vi "ExSubNframeColAdvDisp.vi"(0 "Handle Cluster":T1, 1 "SITKFULLDISPLAYLib.SITKFullDisplay":refnum<k7>, 2 "Number of Images":u32=1 min=1 step=1, 3 "error in (no error)":errorcluster) -> (4 "Handle Cluster":T1, 5 "error out":errorcluster)   [LabVIEW 2010]
panel:
  # "ExSubNframeColAdvDisp:\nThis is a sub VI that collects N frames from the camera\nsystem. This assumes camera has been setup and \ninitialized and that the start camera is done. It also \nassumes the camera has circular buffer capabillities.\nThis is not true for all cameras."
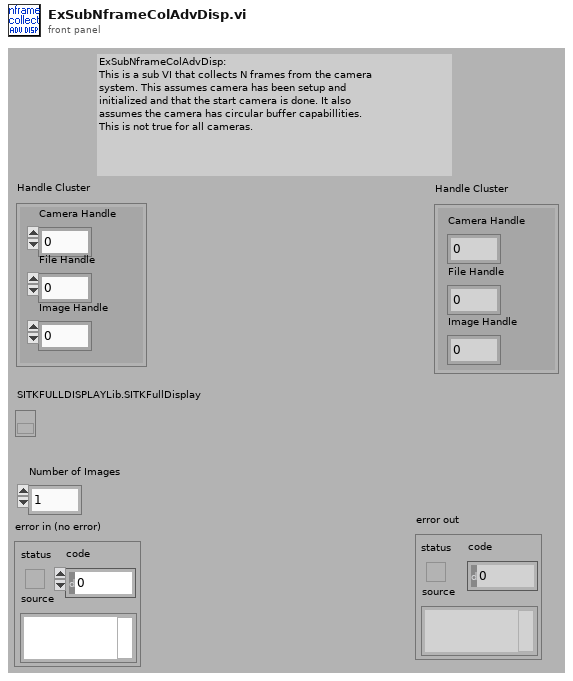
[diagram p1: front panel]
types:
  T1 = cluster{"Camera Handle":u32, "File Handle":u32, "Image Handle":u32}
  T2 = cluster{i32, "X dimension":u32, i32, "Y dimension":u32}
  T3 = cluster{"Min Value":dbl, "Min X Pos":u32, "Min Y Pos":u32, "Max Value":dbl, "Max X Pos":u32, "Max Y Pos":u32, "Reserved 1":dbl, "Reserved2":u32, "Reserved3":u32, "Mean Value":dbl, "StdDev":dbl, "Variance":dbl, "Centroid X":dbl, "Centroid Y":dbl, "Total Area":dbl}
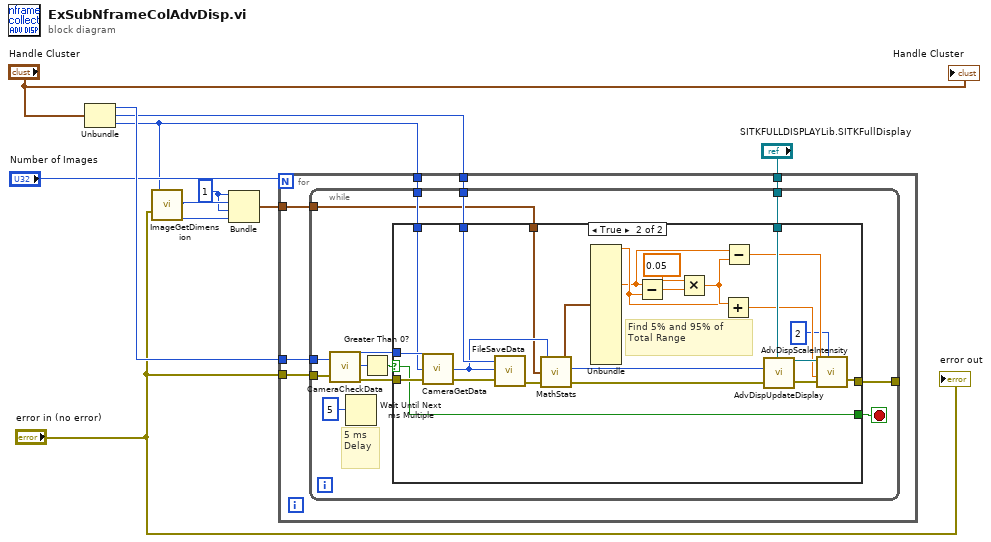
[diagram p0: block diagram]
diagram:
  w1 = 1
  n1 = Unbundle("Handle Cluster") -> ("Camera Handle"=w11:u32, "File Handle"=w6:u32, "Image Handle"=w5:u32)
  n2 = call <userlib>:"ImageGetDimension.vi"("Image Handle"=w5, "error in"="error in (no error)") -> ("X dimension"=w2:u32, "Y dimension"=w7:u32)  [unwired: 4 out]
  n3 = Bundle(w1, "X dimension"=w2, w1, "Y dimension"=w7) -> (w3:T2)  [unwired: 1 in]
  n4 = for {
    N: "Number of Images" -> [_]
    tunnel: w11 -> [w17]
    tunnel: "error in (no error)" -> [w16]
    tunnel: w5 -> [w15]
    tunnel: "SITKFULLDISPLAYLib.SITKFullDisplay" -> [w14]
    tunnel: w6 -> [w13]
    tunnel: w3 -> [w12]
    n5 = while {
      tunnel: w16 -> [w29]
      tunnel: w17 -> [w28]
      tunnel: [w23] -> _
      tunnel: w13 -> [w22]
      tunnel: w15 -> [w21]
      tunnel: w14 -> [w19]
      tunnel: w12 -> [w18]
      stop <- w24 stop-if-true
      # "5 ms\nDelay"
      n6 = call <userlib>:"CameraCheckData.vi"("Camera Handle"=w28, "error in"=w29) -> ("Camera Handle"=w26:u32, "Number Of Frames Available"=w30:i32, "error out"=w25:errorcluster)
      n7 = Wait Until Next ms Multiple(millisecond multiple=5) -> ()  [unwired: 1 out]
      n8 = Greater Than 0?(x=w30) -> (x > 0?=w27:bool)
      n9 = case shown="True" w27 {
        selector: w27 -> [w31 w54]
        tunnel: w26 -> [_ w56]
        tunnel: w25 -> [w32 w55]
        tunnel: [w31 w54] -> w24
        tunnel: [w32 w48] -> w23
        tunnel: w22 -> [_ w52]
        tunnel: w21 -> [_ w51]
        tunnel: w19 -> [_ w50]
        tunnel: w18 -> [_ w41]
        frame False {
        }
        frame True {
          # "Find 5% and 95% of Total Range"
          n10 = call <userlib>:"CameraGetData.vi"("error in"=w55, "Data Handle"=w51, "Camera Handle"=w56) -> ("error out"=w53:errorcluster, "Data Handle"=w43:u32)  [unwired: 1 out]
          n11 = call <userlib>:"FileSaveData.vi"("error in"=w53, "Image Handle"=w43, "File Handle"=w52) -> ("error out"=w42:errorcluster)  [unwired: 1 out]
          n12 = call <userlib>:"MathStats.vi"("error in (no error)"=w42, "Region Of Interest bundle"=w41, "Data Handle"=w43) -> ("error out"=w39:errorcluster, "Statistics Bundle"=w47:T3, "Data Handle"=w40:u32)
          n13 = Unbundle(w47) -> ("Min Value"=w35:dbl, "Max Value"=w34:dbl)  [unwired: 13 out]
          n14 = Subtract(x=w34, y=w35) -> (x-y=w45:dbl)
          n15 = Multiply(x=0.05, y=w45) -> (x*y=w44:dbl)
          n16 = Add(x=w35, y=w44) -> (x+y=w37:dbl)
          n17 = Subtract(x=w34, y=w44) -> (x-y=w36:dbl)
          n18 = call <userlib>:"AdvDispUpdateDisplay.vi"("error in (no error)"=w39, "Image Handle"=w40, "SITKFULLDISPLAYLib.SITKFullDisplay"=w50) -> ("error out"=w38:errorcluster, "SITKFULLDISPLAYLib.SITKFullDisplay"=w49:refnum<k7>)  [unwired: 1 in]
          n19 = call <userlib>:"AdvDispScaleIntensity.vi"("SITKFULLDISPLAYLib.SITKFullDisplay"=w49, "High Intensity"=w36, "Low Intensity"=w37, "error in (no error)"=w38, "Type of Scale"=2) -> ("error out"=w48:errorcluster)  [unwired: 1 out]
        }
      }
    }
  }
  "error out" <- "error in (no error)"
  "Handle Cluster" <- "Handle Cluster"
